vi "construct.vi"(8 "error in (no error)":errorcluster, 9 "configuration name":string, 10 "load config file?":bool=TRUE, 11 "DAQ_DL091205Readers in":refnum<class "DAQ_DL091205Readers.lvclass">) -> (0 "error out":errorcluster, 3 "DAQ_DL091205Readers out":refnum<class "DAQ_DL091205Readers.lvclass">)   [LabVIEW 2010, in "DAQ_DL091205Readers.lvclass"]
uses:
  DAQ_DL091205Readers.lvclass
  DAQ_DL090211Scaffold/DAQ_DL090211Scaffold/DAQ_DL090211Scaffold.lvclass
  SignalReader/GenericSignalReader/GenericSignalReader/GenericSignalReader.lvclass
  DAQ_DL091205Readers.lvclass/DAQ_DL091205Readers.ctl
  common/classes/ErrorController/ErrorController/class_data.vi
  common/classes/GenericComponent/GenericComponent/GenericComponent.lvclass
  common/classes/ErrorController/ErrorController/ErrorController.lvclass
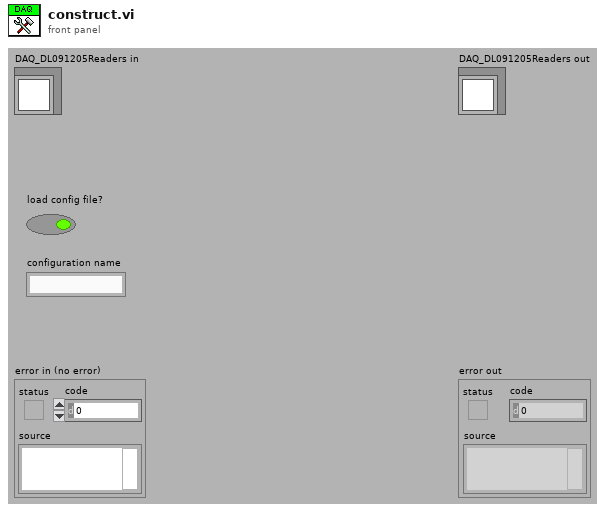
[diagram p1: front panel]
types:
  T1 = typedef "plugin_specification.ctl" = cluster{"class path":string, "configuration":string, "label":string, "settings name":string}
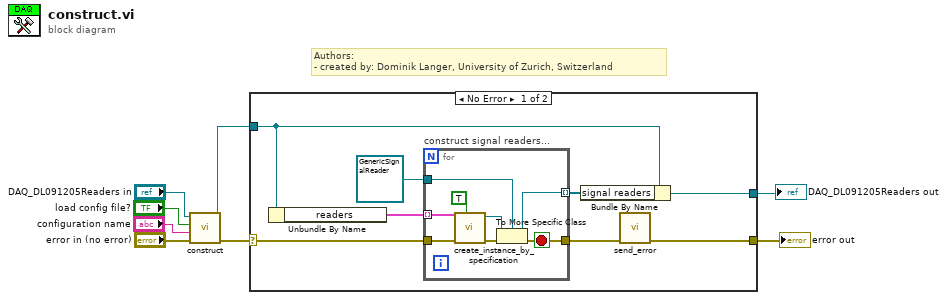
[diagram p0: block diagram]
diagram:
  # "Authors: \n- created by: Dominik Langer, University of Zurich, Switzerland"
  n1 = call-parent "construct.vi"("error in (no error)"="error in (no error)", "configuration name"="configuration name", "load config file?"="load config file?", "GenericPlugin in"="DAQ_DL091205Readers in") -> ("error out"=w4:errorcluster, "GenericPlugin out"=w3:refnum<class "DAQ_DL091205Readers.lvclass">)  [unwired: 6 in]
  n2 = case shown="No Error" w4 {
    selector: w4 -> [w16 w25]
    tunnel: w3 -> [w14 w26]
    tunnel: [w9 w25] -> w1
    tunnel: [w11 w26] -> w2
    frame No Error {
      n3 = Unbundle By Name(w14) -> ("readers"=w15:T1[])
      n4 = for "construct signal readers..." {
        tunnel: w15 -> [w23] mode=indexing
        tunnel: [w19] -> w13 mode=indexing
        tunnel: refnum<class "GenericSignalReader.lvclass"> refnum ("GenericSignalReader.lvclass") -> [w22]
        tunnel: w16 -> [w24]
        tunnel: [w17] -> w10
        stop <- w17 stop-if-true
        n5 = call "create_instance_by_specification.vi"("call constructor?"=TRUE, "error in (no error)"=w24, "component specification"=w23) -> ("error out"=w21:errorcluster, "GenericPlugin out"=w20:refnum<class "GenericComponent.lvclass">)  [unwired: 6 in, 1 out]
        n6 = To More Specific Class(target class=w22, reference=w20, error in=w21) -> (specific class reference=w19:refnum<class "GenericSignalReader.lvclass">, error out=w17:errorcluster)
      }
      n7 = Bundle By Name(cluster=w14, "signal readers"=w13) -> (w11:refnum<class "DAQ_DL091205Readers.lvclass">)
      n8 = call "send_error.vi"("error in (no error)"=w10) -> ("error out"=w9:errorcluster)  [unwired: 10 in]
    }
    frame Error {
    }
  }
  "error out" <- w1
  "DAQ_DL091205Readers out" <- w2
